vi "ti2_setZPos.vi"(8 "error in (no error)":errorcluster, 11 "z Position (um)":dbl) -> (0 "error out":errorcluster)   [LabVIEW 2018, in "ti2lv.lvlib"]
uses:
  ti2lv.lvlib
  ti2wrap/x64/Release/ti2wrap.dll
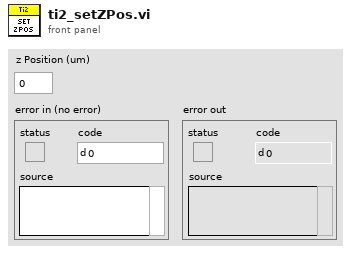
[diagram p1: front panel]
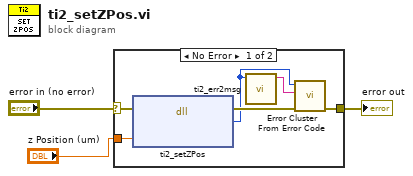
[diagram p0: block diagram]
diagram:
  n1 = case shown="No Error" "error in (no error)" {
    selector: "error in (no error)" -> [w8 w10]
    tunnel: [w9 w10] -> w3
    tunnel: "z Position (um)" -> [w4 _]
    frame No Error {
      n2 = dll-call lib="C:/LVCUR/Flash Gordon v0.6.1b/Hardware/Ti2/ti2wrap/x64/Release/ti2wrap.dll" fn="ti2_setZPos"(error in=w8, "zPos_um"=w4) -> (error out=w7:errorcluster, "return type"=w6:i32)  [unwired: 3 in, 1 out]
      n3 = call "ti2_err2msg.vi"("Error Code"=w6) -> ("Error Message"=w5:string)  [unwired: 10 in]
      n4 = call <vilib>:"Error Cluster From Error Code.vi"("error in (no error)"=w7, "error message (\"\")"=w5, "error code (0)"=w6) -> ("error out"=w9:errorcluster)  [unwired: 6 in]
    }
    frame Error {
    }
  }
  "error out" <- w3
